vi "Configure AM Enabled [AM] Core.vi"(8 "error in (no error)":errorcluster, 9 "AM enabled (True)":bool=TRUE, 10 "Channel Name (\"\")":string="CHANNEL1" caption="channel name (\"CHANNEL1\")", 11 "CS++Fgen in":refnum<class "CS++Fgen.lvclass">) -> (0 "error out":errorcluster, 3 "CS++Fgen out":refnum<class "CS++Fgen.lvclass">)   [LabVIEW 2013, in "CS++Fgen.lvlib" / "CS++Fgen.lvclass"]
doc: "This VI configures whether the function generator applies amplitude modulation to the channel.\n\nNotes:\n\n(1) This VI is part of the IviFgenModulateAM [AM] extension group."
uses:
  CS++Fgen.lvclass
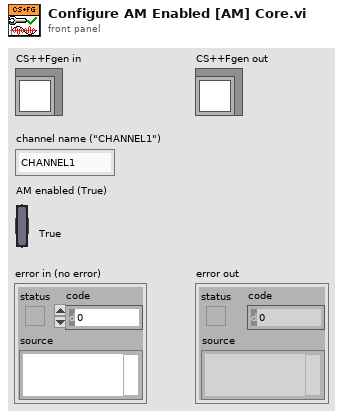
[diagram p1: front panel]
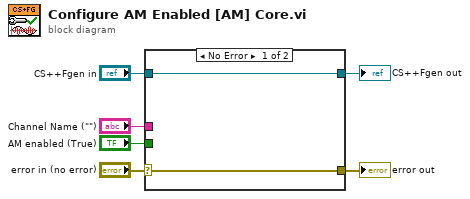
[diagram p0: block diagram]
diagram:
  n1 = case shown="No Error" "error in (no error)" {
    selector: "error in (no error)" -> [w7 w10]
    tunnel: [w7 w10] -> w5
    tunnel: [w8 w9] -> w3
    tunnel: "CS++Fgen in" -> [w8 w9]
    tunnel: "Channel Name (\"\")" -> [_ _]
    tunnel: "AM enabled (True)" -> [_ _]
    frame No Error {
    }
    frame Error {
    }
  }
  "error out" <- w5
  "CS++Fgen out" <- w3
